vi "measure-6221-SR830(SubVI).vi"(0 "输入簇":T1={"initialize"=enum."SR830", "6221"={"6221 Resource"="GPIB0::24::INSTR", "Delta status"=FALSE, "电流|RMS(A)"=0.0}, "SR830+6221"={"source"=0, "Current(A)"=0.0, "阻抗(Ohm)"=0.0, "SR830 1"=FALSE, "SR830 2"=FALSE, "SR830 3"=FALSE, "SR830 4"=FALSE, "VISA 1"="", "VISA 2"="", "VISA 3"="", "VISA 4"="", "Reserve 1"=0, "Reserve 2"=-1, "Reserve 3"=-1, "Reserve 4"=-1, "Sensitivity 1"=-1, "Sensitivity 2"=0, "Sensitivity 3"=-1, "Sensitivity 4"=-1, "量程入 1"=0, "量程入 2"=0, "量程入 3"=0, "量程入 4"=0}, "2400"={"2400"=FALSE, "VISA"="", "Output Level (0)"=1e-05, "Compliance  Level (0.1)"=10.0}, "ch"={"ch"=[], "current"=[], "change?"=[], "holding current\nwhen change ch?"=FALSE}, "Instrument"={"325 Resource "="GPIB0::13::INSTR", "Input (0:A) 325"=0, "Heater Output (1:1) 325"=1, "340 Resource"="GPIB0::14::INSTR", "Input (0:A) 340"=0, "Loop (0: 1)"=0, "Input (0:B) 340"=1, "Loop (1: 1)"=0, "340 Status"=refnum, "Instrument Type"=enum."PPMS-Rotate", "quantum design"=refnum, "semaphore 325"=refnum, "TCP master instance"=refnum, "M24C Resource"="GPIB0::24::INSTR", "4G supply"="GPIB0::24::INSTR", "Temp Status 24C"=refnum, "Temp"=refnum, "9T信号"=refnum, "limit"={"Field limit"=0.0, "Field rate limit"=0.0, "Temp limit"=0.0, "Temp low limit"=0.0, "Temp rate limit "=0.0}, "4g supply status"=refnum, "vi路径"="", "in-plane"="", "out-plane"="", "in-plane signal"=FALSE, "out-plane signal"=FALSE, "in plane 信号"=refnum, "pzt volt"=refnum, "Aborting"=refnum, "数据文件"=refnum, "warning"=refnum, "750 visa"="", "750 rotate"="", "335 Status 2"=refnum, "335 Resource "="GPIB0::24::INSTR", "Input (0:A) 335"=0, "Input (0:B) 335"=1, "Heater Output (1:1) 335"=1, "semaphore 340"=refnum, "semaphore 335"=refnum, "325 Status"=refnum, "semaphore 750"=refnum, "750 field status"=refnum, "camg 振荡状态"=refnum, "列表框"=refnum, "编辑列表框？"=refnum, "camg Rate"=refnum, "行数"=refnum}, "2614B"={"2614B chA"=FALSE, "2614B chB"=FALSE, "VISA"=""}, "33522b"={"33522b resource name"="", "零电压"=0.0, "最大电压"=148.0, "间隔"=4.0, "最小电压"=-48.0, "PZT Scan?"=FALSE}, "gating type"=enum."2614(daul)", "层数"=0, "行数"=0, "是否处理"=[]} {"Instrument"."Loop (1: 1)" items=["1"=1, "2"=2]; "Instrument"."Loop (0: 1)" items=["1"=1, "2"=2]; "Instrument"."Input (0:B) 340" items=["A", "B", "C", "D"]; "Instrument"."Heater Output (1:1) 335" items=["1"=1, "2"=2]; "Instrument"."Input (0:B) 335" items=["A", "B"]; "Instrument"."Input (0:A) 335" items=["A", "B"]; "Instrument"."Heater Output (1:1) 325" items=["1"=1, "2"=2]; "Instrument"."Input (0:A) 325" items=["A", "B"]; "Instrument"."Input (0:A) 340" items=["1"=1, "2"=2]; "SR830+6221"."Sensitivity 4" items=["Auto Gain"=-1, "2 nV/fA"=0, "5 nV/fA"=1, "10 nV/fA"=2, "20 nV/fA"=3, "50 nV/fA"=4, "100 nV/fA"=5, "200 nV/fA"=6, "500 nV/fA"=7, "1 uV/pA"=8, "2 uV/pA"=9, "5 uV/pA"=10, "10 uV/pA"=11, "20 uV/pA"=12, "50 uV/pA"=13, "100 uV/pA"=14, "200 uV/pA"=15, "500 uV/pA"=16, "1 mV/nA"=17, "2 mV/nA"=18, "5 mV/nA"=19, "10 mV/nA"=20, "20 mV/nA"=21, "50 mV/nA"=22, "100 mV/nA"=23, "200 mV/nA"=24, "500 mV/mA"=25, "1 V/uA"=26]; "SR830+6221"."Sensitivity 3" items=["Auto Gain"=-1, "2 nV/fA"=0, "5 nV/fA"=1, "10 nV/fA"=2, "20 nV/fA"=3, "50 nV/fA"=4, "100 nV/fA"=5, "200 nV/fA"=6, "500 nV/fA"=7, "1 uV/pA"=8, "2 uV/pA"=9, "5 uV/pA"=10, "10 uV/pA"=11, "20 uV/pA"=12, "50 uV/pA"=13, "100 uV/pA"=14, "200 uV/pA"=15, "500 uV/pA"=16, "1 mV/nA"=17, "2 mV/nA"=18, "5 mV/nA"=19, "10 mV/nA"=20, "20 mV/nA"=21, "50 mV/nA"=22, "100 mV/nA"=23, "200 mV/nA"=24, "500 mV/mA"=25, "1 V/uA"=26]; "SR830+6221"."Sensitivity 1" items=["Auto Gain"=-1, "2 nV/fA"=0, "5 nV/fA"=1, "10 nV/fA"=2, "20 nV/fA"=3, "50 nV/fA"=4, "100 nV/fA"=5, "200 nV/fA"=6, "500 nV/fA"=7, "1 uV/pA"=8, "2 uV/pA"=9, "5 uV/pA"=10, "10 uV/pA"=11, "20 uV/pA"=12, "50 uV/pA"=13, "100 uV/pA"=14, "200 uV/pA"=15, "500 uV/pA"=16, "1 mV/nA"=17, "2 mV/nA"=18, "5 mV/nA"=19, "10 mV/nA"=20, "20 mV/nA"=21, "50 mV/nA"=22, "100 mV/nA"=23, "200 mV/nA"=24, "500 mV/mA"=25, "1 V/uA"=26]; "SR830+6221"."Sensitivity 2" items=["Auto Gain"=-1, "2 nV/fA"=0, "5 nV/fA"=1, "10 nV/fA"=2, "20 nV/fA"=3, "50 nV/fA"=4, "100 nV/fA"=5, "200 nV/fA"=6, "500 nV/fA"=7, "1 uV/pA"=8, "2 uV/pA"=9, "5 uV/pA"=10, "10 uV/pA"=11, "20 uV/pA"=12, "50 uV/pA"=13, "100 uV/pA"=14, "200 uV/pA"=15, "500 uV/pA"=16, "1 mV/nA"=17, "2 mV/nA"=18, "5 mV/nA"=19, "10 mV/nA"=20, "20 mV/nA"=21, "50 mV/nA"=22, "100 mV/nA"=23, "200 mV/nA"=24, "500 mV/mA"=25, "1 V/uA"=26]; "SR830+6221"."Reserve 4" items=["Auto Gain"=-1, "2 nV/fA"=0, "5 nV/fA"=1, "10 nV/fA"=2, "20 nV/fA"=3, "50 nV/fA"=4, "100 nV/fA"=5, "200 nV/fA"=6, "500 nV/fA"=7, "1 uV/pA"=8, "2 uV/pA"=9, "5 uV/pA"=10, "10 uV/pA"=11, "20 uV/pA"=12, "50 uV/pA"=13, "100 uV/pA"=14, "200 uV/pA"=15, "500 uV/pA"=16, "1 mV/nA"=17, "2 mV/nA"=18, "5 mV/nA"=19, "10 mV/nA"=20, "20 mV/nA"=21, "50 mV/nA"=22, "100 mV/nA"=23, "200 mV/nA"=24, "500 mV/mA"=25, "1 V/uA"=26]; "SR830+6221"."Reserve 3" items=["Auto Reserve"=-1, "High Reserve"=0, "Normal"=1, "Low Noise"=2]; "SR830+6221"."Reserve 2" items=["Auto Reserve"=-1, "High Reserve"=0, "Normal"=1, "Low Noise"=2]; "SR830+6221"."Reserve 1" items=["Auto Reserve"=-1, "High Reserve"=0, "Normal"=1, "Low Noise"=2]; "SR830+6221"."source" items=["SR830 1", "SR830 2", "SR830 3", "SR830 4"]}, 11 "错误输入":errorcluster) -> (4 "输出数组":string[](array[string]), 6 "输出簇":T1={"initialize"=enum."SR830", "6221"={"6221 Resource"="GPIB0::24::INSTR", "Delta status"=FALSE, "电流|RMS(A)"=0.0}, "SR830+6221"={"source"=0, "Current(A)"=0.0, "阻抗(Ohm)"=0.0, "SR830 1"=FALSE, "SR830 2"=FALSE, "SR830 3"=FALSE, "SR830 4"=FALSE, "VISA 1"="", "VISA 2"="", "VISA 3"="", "VISA 4"="", "Reserve 1"=0, "Reserve 2"=-1, "Reserve 3"=-1, "Reserve 4"=-1, "Sensitivity 1"=-1, "Sensitivity 2"=0, "Sensitivity 3"=-1, "Sensitivity 4"=-1, "量程入 1"=0, "量程入 2"=0, "量程入 3"=0, "量程入 4"=0}, "2400"={"2400"=FALSE, "VISA"="", "Output Level (0)"=1e-05, "Compliance  Level (0.1)"=10.0}, "ch"={"ch"=[], "current"=[], "change?"=[], "holding current\nwhen change ch?"=FALSE}, "Instrument"={"325 Resource "="GPIB0::13::INSTR", "Input (0:A) 325"=0, "Heater Output (1:1) 325"=1, "340 Resource"="GPIB0::14::INSTR", "Input (0:A) 340"=0, "Loop (0: 1)"=0, "Input (0:B) 340"=1, "Loop (1: 1)"=0, "340 Status"=refnum, "Instrument Type"=enum."PPMS-Rotate", "quantum design"=refnum, "semaphore 325"=refnum, "TCP master instance"=refnum, "M24C Resource"="GPIB0::24::INSTR", "4G supply"="GPIB0::24::INSTR", "Temp Status 24C"=refnum, "Temp"=refnum, "9T信号"=refnum, "limit"={"Field limit"=0.0, "Field rate limit"=0.0, "Temp limit"=0.0, "Temp low limit"=0.0, "Temp rate limit "=0.0}, "4g supply status"=refnum, "vi路径"="", "in-plane"="", "out-plane"="", "in-plane signal"=FALSE, "out-plane signal"=FALSE, "in plane 信号"=refnum, "pzt volt"=refnum, "Aborting"=refnum, "数据文件"=refnum, "warning"=refnum, "750 visa"="", "750 rotate"="", "335 Status 2"=refnum, "335 Resource "="GPIB0::24::INSTR", "Input (0:A) 335"=0, "Input (0:B) 335"=1, "Heater Output (1:1) 335"=1, "semaphore 340"=refnum, "semaphore 335"=refnum, "325 Status"=refnum, "semaphore 750"=refnum, "750 field status"=refnum, "camg 振荡状态"=refnum, "列表框"=refnum, "编辑列表框？"=refnum, "camg Rate"=refnum, "行数"=refnum}, "2614B"={"2614B chA"=FALSE, "2614B chB"=FALSE, "VISA"=""}, "33522b"={"33522b resource name"="", "零电压"=0.0, "最大电压"=148.0, "间隔"=4.0, "最小电压"=-48.0, "PZT Scan?"=FALSE}, "gating type"=enum."2614(daul)", "层数"=0, "行数"=0, "是否处理"=[]} {"Instrument"."Loop (1: 1)" items=["1"=1, "2"=2]; "Instrument"."Loop (0: 1)" items=["1"=1, "2"=2]; "Instrument"."Input (0:B) 340" items=["A", "B", "C", "D"]; "Instrument"."Heater Output (1:1) 335" items=["1"=1, "2"=2]; "Instrument"."Input (0:B) 335" items=["A", "B"]; "Instrument"."Input (0:A) 335" items=["A", "B"]; "Instrument"."Heater Output (1:1) 325" items=["1"=1, "2"=2]; "Instrument"."Input (0:A) 325" items=["A", "B"]; "Instrument"."Input (0:A) 340" items=["1"=1, "2"=2]; "SR830+6221"."Sensitivity 4" items=["Auto Gain"=-1, "2 nV/fA"=0, "5 nV/fA"=1, "10 nV/fA"=2, "20 nV/fA"=3, "50 nV/fA"=4, "100 nV/fA"=5, "200 nV/fA"=6, "500 nV/fA"=7, "1 uV/pA"=8, "2 uV/pA"=9, "5 uV/pA"=10, "10 uV/pA"=11, "20 uV/pA"=12, "50 uV/pA"=13, "100 uV/pA"=14, "200 uV/pA"=15, "500 uV/pA"=16, "1 mV/nA"=17, "2 mV/nA"=18, "5 mV/nA"=19, "10 mV/nA"=20, "20 mV/nA"=21, "50 mV/nA"=22, "100 mV/nA"=23, "200 mV/nA"=24, "500 mV/mA"=25, "1 V/uA"=26]; "SR830+6221"."Sensitivity 3" items=["Auto Gain"=-1, "2 nV/fA"=0, "5 nV/fA"=1, "10 nV/fA"=2, "20 nV/fA"=3, "50 nV/fA"=4, "100 nV/fA"=5, "200 nV/fA"=6, "500 nV/fA"=7, "1 uV/pA"=8, "2 uV/pA"=9, "5 uV/pA"=10, "10 uV/pA"=11, "20 uV/pA"=12, "50 uV/pA"=13, "100 uV/pA"=14, "200 uV/pA"=15, "500 uV/pA"=16, "1 mV/nA"=17, "2 mV/nA"=18, "5 mV/nA"=19, "10 mV/nA"=20, "20 mV/nA"=21, "50 mV/nA"=22, "100 mV/nA"=23, "200 mV/nA"=24, "500 mV/mA"=25, "1 V/uA"=26]; "SR830+6221"."Sensitivity 1" items=["Auto Gain"=-1, "2 nV/fA"=0, "5 nV/fA"=1, "10 nV/fA"=2, "20 nV/fA"=3, "50 nV/fA"=4, "100 nV/fA"=5, "200 nV/fA"=6, "500 nV/fA"=7, "1 uV/pA"=8, "2 uV/pA"=9, "5 uV/pA"=10, "10 uV/pA"=11, "20 uV/pA"=12, "50 uV/pA"=13, "100 uV/pA"=14, "200 uV/pA"=15, "500 uV/pA"=16, "1 mV/nA"=17, "2 mV/nA"=18, "5 mV/nA"=19, "10 mV/nA"=20, "20 mV/nA"=21, "50 mV/nA"=22, "100 mV/nA"=23, "200 mV/nA"=24, "500 mV/mA"=25, "1 V/uA"=26]; "SR830+6221"."Sensitivity 2" items=["Auto Gain"=-1, "2 nV/fA"=0, "5 nV/fA"=1, "10 nV/fA"=2, "20 nV/fA"=3, "50 nV/fA"=4, "100 nV/fA"=5, "200 nV/fA"=6, "500 nV/fA"=7, "1 uV/pA"=8, "2 uV/pA"=9, "5 uV/pA"=10, "10 uV/pA"=11, "20 uV/pA"=12, "50 uV/pA"=13, "100 uV/pA"=14, "200 uV/pA"=15, "500 uV/pA"=16, "1 mV/nA"=17, "2 mV/nA"=18, "5 mV/nA"=19, "10 mV/nA"=20, "20 mV/nA"=21, "50 mV/nA"=22, "100 mV/nA"=23, "200 mV/nA"=24, "500 mV/mA"=25, "1 V/uA"=26]; "SR830+6221"."Reserve 4" items=["Auto Gain"=-1, "2 nV/fA"=0, "5 nV/fA"=1, "10 nV/fA"=2, "20 nV/fA"=3, "50 nV/fA"=4, "100 nV/fA"=5, "200 nV/fA"=6, "500 nV/fA"=7, "1 uV/pA"=8, "2 uV/pA"=9, "5 uV/pA"=10, "10 uV/pA"=11, "20 uV/pA"=12, "50 uV/pA"=13, "100 uV/pA"=14, "200 uV/pA"=15, "500 uV/pA"=16, "1 mV/nA"=17, "2 mV/nA"=18, "5 mV/nA"=19, "10 mV/nA"=20, "20 mV/nA"=21, "50 mV/nA"=22, "100 mV/nA"=23, "200 mV/nA"=24, "500 mV/mA"=25, "1 V/uA"=26]; "SR830+6221"."Reserve 3" items=["Auto Reserve"=-1, "High Reserve"=0, "Normal"=1, "Low Noise"=2]; "SR830+6221"."Reserve 2" items=["Auto Reserve"=-1, "High Reserve"=0, "Normal"=1, "Low Noise"=2]; "SR830+6221"."Reserve 1" items=["Auto Reserve"=-1, "High Reserve"=0, "Normal"=1, "Low Noise"=2]; "SR830+6221"."source" items=["SR830 1", "SR830 2", "SR830 3", "SR830 4"]}, 8 "错误输出":errorcluster)   [LabVIEW 2019, in "SubVI.lvlib"]
uses:
  SubVI.lvlib
  ctl/config.ctl
  <vilib>/NI/Modbus Library/API/Master/Modbus Master.lvclass
  ctl/initialize.ctl
  ctl/Instrument.ctl
  ctl/335 state.ctl
  ctl/Instrument Type.ctl
  lib/QDInstrument.dll
  ctl/limit.ctl
  ctl/9T mag field stauts.ctl
  ctl/warning.ctl
  ctl/Gating type.ctl
  lib/Stanford Research 830/Public/Data/Read (All Parameters).vi
  lib/Stanford Research 830/Stanford Research 830.lvlib
  lib/Keithley 622x/Keithley 622x.lvlib
  Get value.lvlib
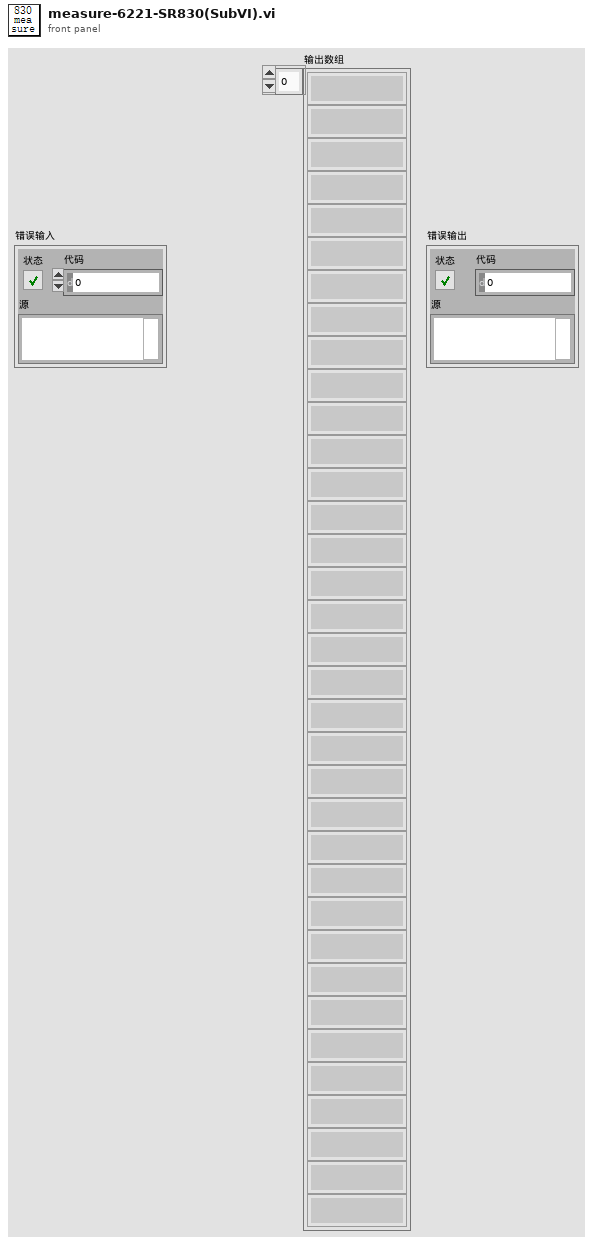
[diagram p1: front panel]
types:
  T1 = typedef "config.ctl" = cluster{"initialize":T2, "6221":cluster{"6221 Resource":refnum<visa-resource-name>, "Delta status":bool, "电流|RMS(A)":dbl}, "SR830+6221":cluster{"source":u16, "Current(A)":dbl, "阻抗(Ohm)":dbl, "SR830 1":bool, "SR830 2":bool, "SR830 3":bool, "SR830 4":bool, "VISA 1":refnum<visa-resource-name>, "VISA 2":refnum<visa-resource-name>, "VISA 3":refnum<visa-resource-name>, "VISA 4":refnum<visa-resource-name>, "Reserve 1":i16, "Reserve 2":i16, "Reserve 3":i16, "Reserve 4":i16, "Sensitivity 1":i16, "Sensitivity 2":i16, "Sensitivity 3":i16, "Sensitivity 4":i16, "量程入 1":i32, "量程入 2":i32, "量程入 3":i32, "量程入 4":i32}, "2400":cluster{"2400":bool, "VISA":refnum<visa-resource-name>, "Output Level (0)":dbl, "Compliance  Level (0.1)":dbl}, "ch":cluster{"ch":i32[], "current":dbl[], "change?":bool[], "holding current\nwhen change ch?":bool}, "Instrument":T3, "2614B":cluster{"2614B chA":bool, "2614B chB":bool, "VISA":refnum<visa-resource-name>}, "33522b":cluster{"33522b resource name":refnum<visa-resource-name>, "零电压":dbl, "最大电压":dbl, "间隔":dbl, "最小电压":dbl, "PZT Scan?":bool}, "gating type":T7, "层数":i32, "行数":i32, "是否处理":bool[]}
  T2 = typedef "initialize.ctl" = enum16{"SR830", "keithley6221-SR830", "Delta", "Delta-tunnelling", "keithley6221-2182-DC", "PZT"}
  T3 = typedef "Instrument.ctl" = cluster{"325 Resource ":refnum<visa-resource-name>, "Input (0:A) 325":u16, "Heater Output (1:1) 325":u16, "340 Resource":refnum<visa-resource-name>, "Input (0:A) 340":u16, "Loop (0: 1)":u16, "Input (0:B) 340":u16, "Loop (1: 1)":u16, "340 Status":refnum<vi>, "Instrument Type":T4, "quantum design":refnum<k24>, "semaphore 325":T5, "TCP master instance":refnum<class "Modbus Master.lvclass">, "M24C Resource":refnum<visa-resource-name>, "4G supply":refnum<visa-resource-name>, "Temp Status 24C":refnum<vi>, "Temp":refnum<vi>, "9T信号":T5, "limit":T6, "4g supply status":refnum<vi>, "vi路径":string, "in-plane":refnum<visa-resource-name>, "out-plane":refnum<visa-resource-name>, "in-plane signal":bool, "out-plane signal":bool, "in plane 信号":T5, "pzt volt":refnum<vi>, "Aborting":refnum<vi>, "数据文件":refnum<vi>, "warning":refnum<vi>, "750 visa":refnum<visa-resource-name>, "750 rotate":refnum<visa-resource-name>, "335 Status 2":refnum<vi>, "335 Resource ":refnum<visa-resource-name>, "Input (0:A) 335":u16, "Input (0:B) 335":u16, "Heater Output (1:1) 335":u16, "semaphore 340":T5, "semaphore 335":T5, "325 Status":refnum<vi>, "semaphore 750":T5, "750 field status":refnum<vi>, "camg 振荡状态":refnum<vi>, "列表框":refnum<vi>, "编辑列表框？":refnum<vi>, "camg Rate":refnum<vi>, "行数":refnum<vi>}
  T4 = typedef "Instrument Type.ctl" = enum16{"PPMS", "VersaLab", "DynaCool", "SVSM", "PPMS-Rotate", "Lakeshore335", "lengtou2", "9T mag", "9T cmag rotate", "test"}
  T5 = typedef "Semaphore RefNum" = refnum<k1>
  T6 = typedef "limit.ctl" = cluster{"Field limit":dbl, "Field rate limit":dbl, "Temp limit":dbl, "Temp low limit":dbl, "Temp rate limit ":dbl}
  T7 = typedef "Gating type.ctl" = enum32{"null", "2614(daul)", "2400"}
  T8 = cluster{"X-Value":dbl, "Y-Value":dbl, "R-Value":dbl, "Theta-Value":dbl, "Aux In 1 Value":dbl, "Aux In 2 Value":dbl, "Aux In 3 Value":dbl, "Aux In 4 Value":dbl, "Reference Frequency":dbl, "Channel 1 Display":dbl, "Channel 2 Display":dbl}
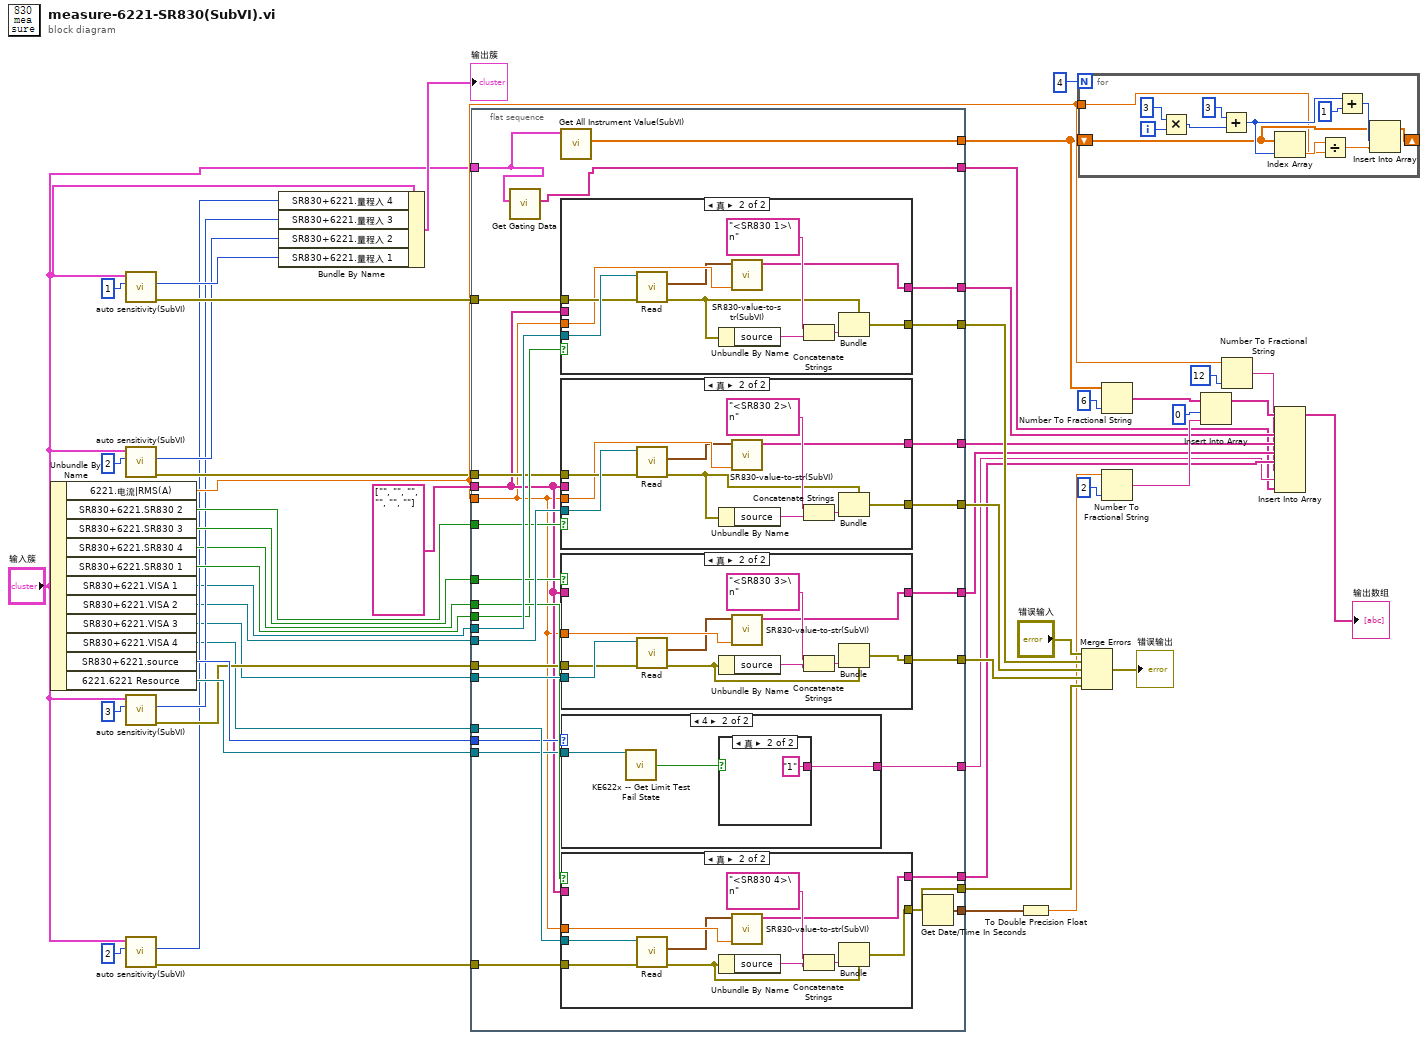
[diagram p0: block diagram]
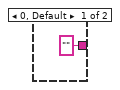
[diagram p2: hidden frame]
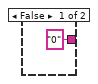
[diagram p3: hidden frame]
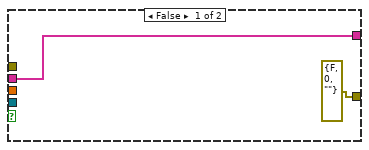
[diagram p4: hidden frame]
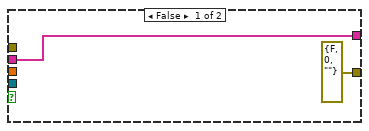
[diagram p5: hidden frame]
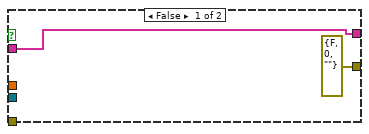
[diagram p6: hidden frame]
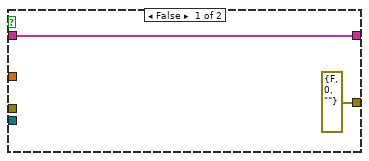
[diagram p7: hidden frame]
diagram:
  n1 = Unbundle By Name("输入簇") -> ("6221.电流|RMS(A)"=w23:dbl, "SR830+6221.SR830 2"=w19:bool, "SR830+6221.SR830 3"=w16:bool, "SR830+6221.SR830 4"=w13:bool, "SR830+6221.SR830 1"=w34:bool, "SR830+6221.VISA 1"=w5:refnum<visa-resource-name>, "SR830+6221.VISA 2"=w4:refnum<visa-resource-name>, "SR830+6221.VISA 3"=w3:refnum<visa-resource-name>, "SR830+6221.VISA 4"=w2:refnum<visa-resource-name>, "SR830+6221.source"=w25:u16, "6221.6221 Resource"=w24:refnum<visa-resource-name>)
  n2 = call "auto sensitivity(SubVI).vi"("SR830 num"=1, "config in"="输入簇") -> ("error out"=w50:errorcluster, "量程"=w43:i32)  [unwired: 8 in]
  n3 = call "auto sensitivity(SubVI).vi"("SR830 num"=2, "config in"="输入簇") -> ("error out"=w18:errorcluster, "量程"=w17:i32)  [unwired: 8 in]
  n4 = call "auto sensitivity(SubVI).vi"("SR830 num"=3, "config in"="输入簇") -> ("error out"=w15:errorcluster, "量程"=w14:i32)  [unwired: 8 in]
  n5 = call "auto sensitivity(SubVI).vi"("SR830 num"=2, "config in"="输入簇") -> ("error out"=w11:errorcluster, "量程"=w12:i32)  [unwired: 8 in]
  n6 = Bundle By Name(cluster="输入簇", "SR830+6221.量程入 4"=w12, "SR830+6221.量程入 3"=w14, "SR830+6221.量程入 2"=w17, "SR830+6221.量程入 1"=w43) -> (→"输出簇":T1)
  n7 = flat-sequence {
    tunnel: [w80] -> w51
    tunnel: w4 -> [w79]
    tunnel: w5 -> [w78]
    tunnel: w2 -> [w77]
    tunnel: w3 -> [w76]
    tunnel: w16 -> [w75]
    tunnel: w13 -> [w74]
    tunnel: w34 -> [w73]
    tunnel: w19 -> [w72]
    tunnel: w50 -> [w71]
    tunnel: w18 -> [w70]
    tunnel: w15 -> [w69]
    tunnel: w11 -> [w68]
    tunnel: [w67] -> w49
    tunnel: [w66] -> w48
    tunnel: [w65] -> w47
    tunnel: [w64] -> w46
    tunnel: [w63] -> w33
    tunnel: [w62] -> w32
    tunnel: [w61] -> w31
    tunnel: w23 -> [w55]
    tunnel: [w60] -> w30
    tunnel: string[] ["", "", "", "", "", ""] ("数组") -> [w56]
    tunnel: [w59] -> w21
    tunnel: w25 -> [w58]
    tunnel: w24 -> [w57]
    tunnel: [w54] -> w22
    tunnel: "输入簇" -> [w53]
    tunnel: [w52] -> w20
    frame #0 {
      n8 = call "Get Gating Data.vi"("簇"=w53) -> ("data"=w52:string[])  [unwired: 10 in]
      n9 = call "Get All Instrument Value(SubVI).vi"("输出簇."=w53) -> ("数组"=w54:dbl[])  [unwired: 10 in]
      n10 = case shown="真" w73 {
        tunnel: w78 -> [_ w110]
        tunnel: w71 -> [_ w109]
        tunnel: [errorcluster {"status"=FALSE, "code"=0, "source"=""} ("error out") w104] -> w67
        tunnel: w55 -> [_ w103]
        tunnel: [w99 w101] -> w63
        tunnel: w56 -> [w99 _]
        frame False {
        }
        frame True {
          n11 = call-poly "Read.vi"("error in (no error)"=w109, "VISA resource name"=w110) -> ("error out"=w105:errorcluster, "Parameter Values"=w102:T8)  [unwired: 7 in, 1 out]
          n12 = Unbundle By Name(w105) -> ("source"=w107:string)
          n13 = call "SR830-value-to-str(SubVI).vi"("电流"=w103, "Parameter Values"=w102) -> ("数组"=w101:string[])  [unwired: 9 in]
          n14 = Concatenate Strings("<SR830 1>\n", w107) -> (w106:string)
          n15 = Bundle(cluster=w105, "source"=w106) -> (w104:errorcluster)  [unwired: 2 in]
        }
      }
      n16 = case shown="真" w72 {
        tunnel: w79 -> [_ w98]
        tunnel: w70 -> [_ w97]
        tunnel: [errorcluster {"status"=FALSE, "code"=0, "source"=""} ("error out") w92] -> w65
        tunnel: w55 -> [_ w91]
        tunnel: [w87 w89] -> w62
        tunnel: w56 -> [w87 _]
        frame False {
        }
        frame True {
          n17 = call-poly "Read.vi"("error in (no error)"=w97, "VISA resource name"=w98) -> ("error out"=w93:errorcluster, "Parameter Values"=w90:T8)  [unwired: 7 in, 1 out]
          n18 = Unbundle By Name(w93) -> ("source"=w95:string)
          n19 = call "SR830-value-to-str(SubVI).vi"("电流"=w91, "Parameter Values"=w90) -> ("数组"=w89:string[])  [unwired: 9 in]
          n20 = Concatenate Strings("<SR830 2>\n", w95) -> (w94:string)
          n21 = Bundle(cluster=w93, "source"=w94) -> (w92:errorcluster)  [unwired: 2 in]
        }
      }
      n22 = case shown="真" w75 {
        tunnel: w76 -> [_ w134]
        tunnel: w69 -> [_ w133]
        tunnel: [errorcluster {"status"=FALSE, "code"=0, "source"=""} ("error out") w128] -> w66
        tunnel: w55 -> [_ w127]
        tunnel: [w123 w125] -> w61
        tunnel: w56 -> [w123 _]
        frame False {
        }
        frame True {
          n23 = call-poly "Read.vi"("error in (no error)"=w133, "VISA resource name"=w134) -> ("error out"=w129:errorcluster, "Parameter Values"=w126:T8)  [unwired: 7 in, 1 out]
          n24 = Unbundle By Name(w129) -> ("source"=w131:string)
          n25 = call "SR830-value-to-str(SubVI).vi"("电流"=w127, "Parameter Values"=w126) -> ("数组"=w125:string[])  [unwired: 9 in]
          n26 = Concatenate Strings("<SR830 3>\n", w131) -> (w130:string)
          n27 = Bundle(cluster=w129, "source"=w130) -> (w128:errorcluster)  [unwired: 2 in]
        }
      }
      n28 = case shown="4" w58 {
        tunnel: ["" w83] -> w59
        tunnel: w57 -> [_ w82]
        frame 0, Default {
        }
        frame 4 {
          n29 = call "KE622x -- Get Limit Test Fail State.vi"("Resource In"=w82) -> ("Limit Test Failed (Compliance)?"=w84:bool)  [unwired: 12 in, 2 out]
          n30 = case shown="真" w84 {
            tunnel: ["0" "1"] -> w83
            frame False {
            }
            frame True {
            }
          }
        }
      }
      n31 = case shown="真" w74 {
        tunnel: w77 -> [_ w122]
        tunnel: w68 -> [_ w121]
        tunnel: [errorcluster {"status"=FALSE, "code"=0, "source"=""} ("error out") w116] -> w64
        tunnel: w55 -> [_ w115]
        tunnel: [w111 w113] -> w60
        tunnel: w56 -> [w111 _]
        frame False {
        }
        frame True {
          n32 = call-poly "Read.vi"("error in (no error)"=w121, "VISA resource name"=w122) -> ("error out"=w117:errorcluster, "Parameter Values"=w114:T8)  [unwired: 7 in, 1 out]
          n33 = Unbundle By Name(w117) -> ("source"=w119:string)
          n34 = call "SR830-value-to-str(SubVI).vi"("电流"=w115, "Parameter Values"=w114) -> ("数组"=w113:string[])  [unwired: 9 in]
          n35 = Concatenate Strings("<SR830 4>\n", w119) -> (w118:string)
          n36 = Bundle(cluster=w117, "source"=w118) -> (w116:errorcluster)  [unwired: 2 in]
        }
      }
      n37 = Get Date/Time In Seconds() -> (seconds since 1Jan1904=w80:timestamp)
    }
  }
  n38 = To Double Precision Float(number=w51) -> (double precision float=w39:dbl)
  n39 = for {
    N: 4 -> [_]
    shift-right: [w143] -> _
    shift-left: w22 -> [w137]
    tunnel: w23 -> [w135]
    i -> [w136]
    n40 = Multiply(x=3, y=w136) -> (x*y=w144:i32)
    n41 = Add(x=3 ("索引"), y=w144) -> (x+y=w142:i32)
    n42 = Index Array(array=w137, index=w142) -> (element=w139:dbl)
    n43 = Divide(x=w139, y=w135) -> (x/y=w138:dbl)
    n44 = Add(x=w142, y=1) -> (x+y=w140:i32)
    n45 = Insert Into Array(array=w137, index=w140, new element=w138) -> (w143:dbl[])
  }
  n46 = Merge Errors("错误输入", w49, w47, w48, w46) -> (→"错误输出":errorcluster)
  n47 = Number To Fractional String(number=w22, precision (6)=i16 6 ("精度(6)")) -> (F-format string=w41:string[])  [unwired: 2 in]
  n48 = Number To Fractional String(number=w39, precision (6)=i16 2 ("精度(6)")) -> (F-format string=w37:string)  [unwired: 2 in]
  n49 = Insert Into Array(array=w41, index=0 ("索引"), new element=w37) -> (w36:string[])
  n50 = Number To Fractional String(number=w23, precision (6)=i16 12 ("精度(6)")) -> (F-format string=w27:string)  [unwired: 2 in]
  n51 = Insert Into Array(array=w36, new element #1=w33, new element #2=w32, new element #3=w31, new element #4=w30, new element #5=w27, new element #6=w21, new element #7=w20) -> (→"输出数组":string[])  [unwired: 1 in]
